vi "GenerateTransmitterCal.vi"(9 "XmitCount":i32, 10 "XmitMin":dbl[](array[numeric]), 11 "XmitMax":dbl[](array[numeric])) -> (2 "TransmitterOffset":string[](array[string]), 3 "TransmitterSlope":string[](array[string]))   [LabVIEW 2010]
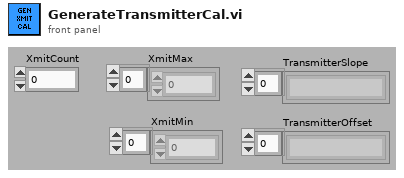
[diagram p1: front panel]
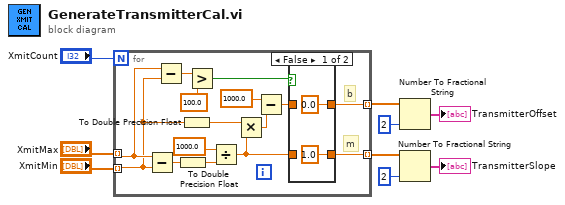
[diagram p0: block diagram]
diagram:
  n1 = for {
    N: "XmitCount" -> [_]
    tunnel: "XmitMin" -> [w13] mode=indexing
    tunnel: "XmitMax" -> [w14] mode=indexing
    tunnel: [w15] -> w9 mode=indexing
    tunnel: [w17] -> w7 mode=indexing
    # "b"
    # "m"
    n2 = Subtract(x=w14, y=w13) -> (x-y=w23:dbl)
    n3 = Subtract(x=w14, y=w13) -> (x-y=w12:dbl)
    n4 = To Double Precision Float(number=w23) -> (double precision float=w22:dbl)
    n5 = To Double Precision Float(number=w13) -> (double precision float=w19:dbl)
    n6 = Greater?(x=w12, y=100.0) -> (0:w10:bool)
    n7 = Divide(x=1000.0, y=w22) -> (x/y=w16:dbl)
    n8 = Multiply(x=w19, y=w16) -> (x*y=w20:dbl)
    n9 = Subtract(x=1000.0, y=w20) -> (x-y=w18:dbl)
    n10 = case shown="False" w10 {
      tunnel: [0.0 w28] -> w17
      tunnel: w18 -> [_ w28]
      tunnel: w16 -> [_ w27]
      tunnel: [1.0 w27] -> w15
      frame False {
      }
      frame True {
      }
    }
  }
  n11 = Number To Fractional String(number=w7, precision (6)=i16 2) -> (F-format string=→"TransmitterOffset":string[])  [unwired: 2 out]
  n12 = Number To Fractional String(number=w9, precision (6)=i16 2) -> (F-format string=→"TransmitterSlope":string[])  [unwired: 2 out]
